vi "Delete.vi"(8 "error in (no error)":errorcluster caption="entrée d'erreur (pas d'erreur)", 11 "Database Drivers en entrée":refnum<class "Database Drivers.lvclass">) -> (0 "error out":errorcluster caption="sortie d'erreur", 3 "Database Drivers en sortie":refnum<class "Database Drivers.lvclass">)   [LabVIEW 2020, in "Library Instrument & Equipement.lvlib" / "Library Database.lvlib" / "Database Drivers.lvclass"]
uses:
  Database Drivers.lvclass
  Database Drivers.lvclass/Database Drivers.ctl
  <vilib>/addons/database/NI_Database_API.lvlib
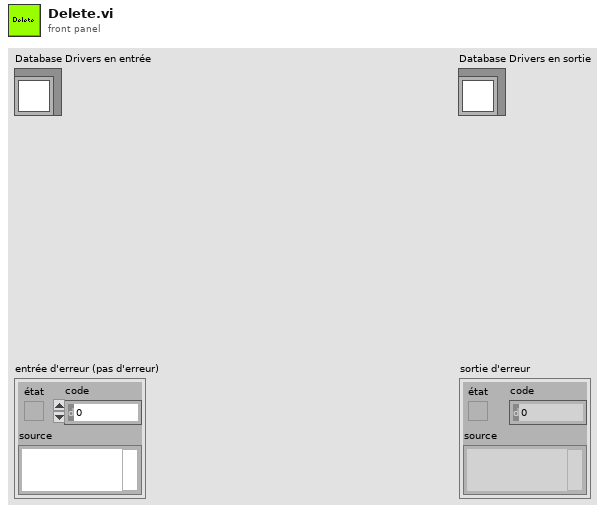
[diagram p1: front panel]
types:
  T1 = typedef "NI_Database_API.lvlib/Conn ObjectReference.ctl" = refnum<k1>
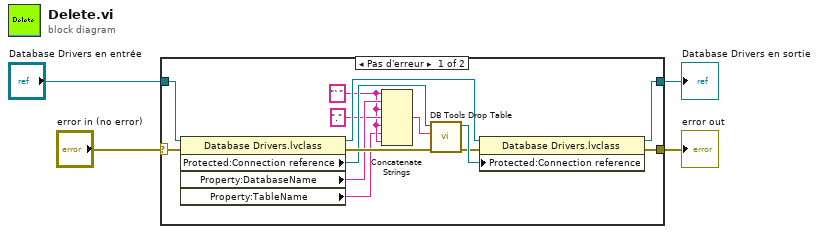
[diagram p0: block diagram]
diagram:
  n1 = case shown="Pas d'erreur" "error in (no error)" {
    selector: "error in (no error)" -> [w11 w20]
    tunnel: [w10 w20] -> w3
    tunnel: [w12 w19] -> w1
    tunnel: "Database Drivers en entrée" -> [w18 w19]
    frame No Error {
      w6 = "`" ("chaîne")
      n2 = property class="Database Drivers.lvclass"(reference=w18, error in=w11) -> (reference out=w13:refnum<class "Database Drivers.lvclass">, error out=w17:errorcluster, "Protected:Connection reference"=w16:T1, "Property:DatabaseName"=w9:string, "Property:TableName"=w5:string)
      n3 = Concatenate Strings(w6, w9, w6, "." ("chaîne"), w6, w5, w6) -> (w8:string)
      n4 = call <vilib>:"DB Tools Drop Table.vi"("error in (no error)"=w17, "table"=w8, "connection reference"=w16) -> ("error out"=w14:errorcluster, "connection reference out"=w15:T1)  [unwired: 5 in]
      n5 = property class="Database Drivers.lvclass"(reference=w13, error in=w14, "Protected:Connection reference"=w15) -> (reference out=w12:refnum<class "Database Drivers.lvclass">, error out=w10:errorcluster)
    }
    frame Error {
    }
  }
  "error out" <- w3
  "Database Drivers en sortie" <- w1
